vi "PathTest.vi"() -> (3 "path":path)   [LabVIEW 2020, in "DriverCommon.lvlib"]
uses:
  DriverCommon.lvlib
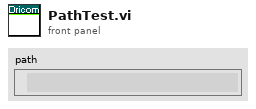
[diagram p1: front panel]
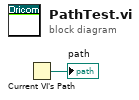
[diagram p0: block diagram]
diagram:
  n1 = Current VI's Path() -> (path=→"path":path)
